vi "CRYCalibration.vi"(4 "O_Signal Type Old In":string[][](array[string]), 5 "Apply?":bool=TRUE, 6 "I_Signal Type Old In":string[][](array[string]), 7 "Hardware In":string, 8 "O_Calibrated Device Name Old In":string[][](array[string]), 9 "I_Calibrated Device Name Old In":string[][](array[string]), 10 "Calibration":T1 {"Calibration 2D"."Sens Curve"."Z data" items=["dB", "Lin"]; "Calibration 2D"."Sens Curve"."X data" items=["dB", "Lin"]; "Calibration 2D"."Sens Curve"."Y data" items=["dB", "Lin"]; "Calibration 2D"."Sens Curve"."Z dB ref" format="%.1f"; "Calibration 2D"."Sens Curve"."Z axis" items=["Log", "Lin"]; "Calibration 2D"."Sens Curve"."X dB ref" format="%.1f"; "Calibration 2D"."Sens Curve"."X axis" items=["Log", "Lin"]; "Calibration 2D"."Sens Curve"."Y axis" items=["Log", "Lin"]; "Calibration 2D"."Sens Curve"."Y dB ref" format="%.1f"; "Calibration 2D"."Sens Curve"."Curve"."z" format="%.2f"; "Calibration 2D"."Sens Curve"."Curve"."y" format="%.5p"; "Calibration 2D"."Sens Curve"."Curve"."x" format="%.2f"; "Calibration 2D"."EQ Curve"."Z data" items=["dB", "Lin"]; "Calibration 2D"."EQ Curve"."X data" items=["dB", "Lin"]; "Calibration 2D"."EQ Curve"."Y data" items=["dB", "Lin"]; "Calibration 2D"."EQ Curve"."Z dB ref" format="%.1f"; "Calibration 2D"."EQ Curve"."Z axis" items=["Log", "Lin"]; "Calibration 2D"."EQ Curve"."X dB ref" format="%.1f"; "Calibration 2D"."EQ Curve"."X axis" items=["Log", "Lin"]; "Calibration 2D"."EQ Curve"."Y axis" items=["Log", "Lin"]; "Calibration 2D"."EQ Curve"."Y dB ref" format="%.1f"; "Calibration 2D"."EQ Curve"."Curve"."z" format="%.2f"; "Calibration 2D"."EQ Curve"."Curve"."y" format="%.2f"; "Calibration 2D"."EQ Curve"."Curve"."x" format="%.2f"; "Calibration 2D"."Corr Curve"."Z data" items=["dB", "Lin"]; "Calibration 2D"."Corr Curve"."X data" items=["dB", "Lin"]; "Calibration 2D"."Corr Curve"."Y data" items=["dB", "Lin"]; "Calibration 2D"."Corr Curve"."Z dB ref" format="%.1f"; "Calibration 2D"."Corr Curve"."Z axis" items=["Log", "Lin"]; "Calibration 2D"."Corr Curve"."X dB ref" format="%.1f"; "Calibration 2D"."Corr Curve"."X axis" items=["Log", "Lin"]; "Calibration 2D"."Corr Curve"."Y axis" items=["Log", "Lin"]; "Calibration 2D"."Corr Curve"."Y dB ref" format="%.1f"; "Calibration 2D"."Corr Curve"."Curve"."z" format="%.2f"; "Calibration 2D"."Corr Curve"."Curve"."y" format="%.2f"; "Calibration 2D"."Corr Curve"."Curve"."x" format="%.2f"; "Calibration 2D"."Calibration"."EQ Step size" items=["R10", "R20", "R40", "R80", "User"]; "Calibration 2D"."Calibration"."Corr Step size" items=["R10", "R20", "R40", "R80", "User"]}, 11 "Proper VI No In":i32) -> (0 "O_Calibrated Device Name Out":string[][](array[string]), 1 "I_Calibrated Device Name Out":string[][](array[string]), 2 "O_Signal Type Out":string[][](array[string]), 3 "I_Signal Type Out":string[][](array[string]))   [LabVIEW 2013]
uses:
  Typedef Control/CRYCalibration All Cluster.ctl
  Typedef Control/CRYCalibration 2DCluster.ctl
  Typedef Control/CRYCalibration Cluster.ctl
  Typedef Control/CRYData Cluster.ctl
  CRYProject/CRYProject Editor Global.vi
panel:
  out "O_Signal Type Old In 2":string[][](array[string])
  out "I_Signal Type Old In 2":string[][](array[string])
  out "O_Name Out(Output Calibrated Name Out)":string[][](array[string])
  out "I_Name Out(Input Calibrated Name Out)":string[][](array[string])
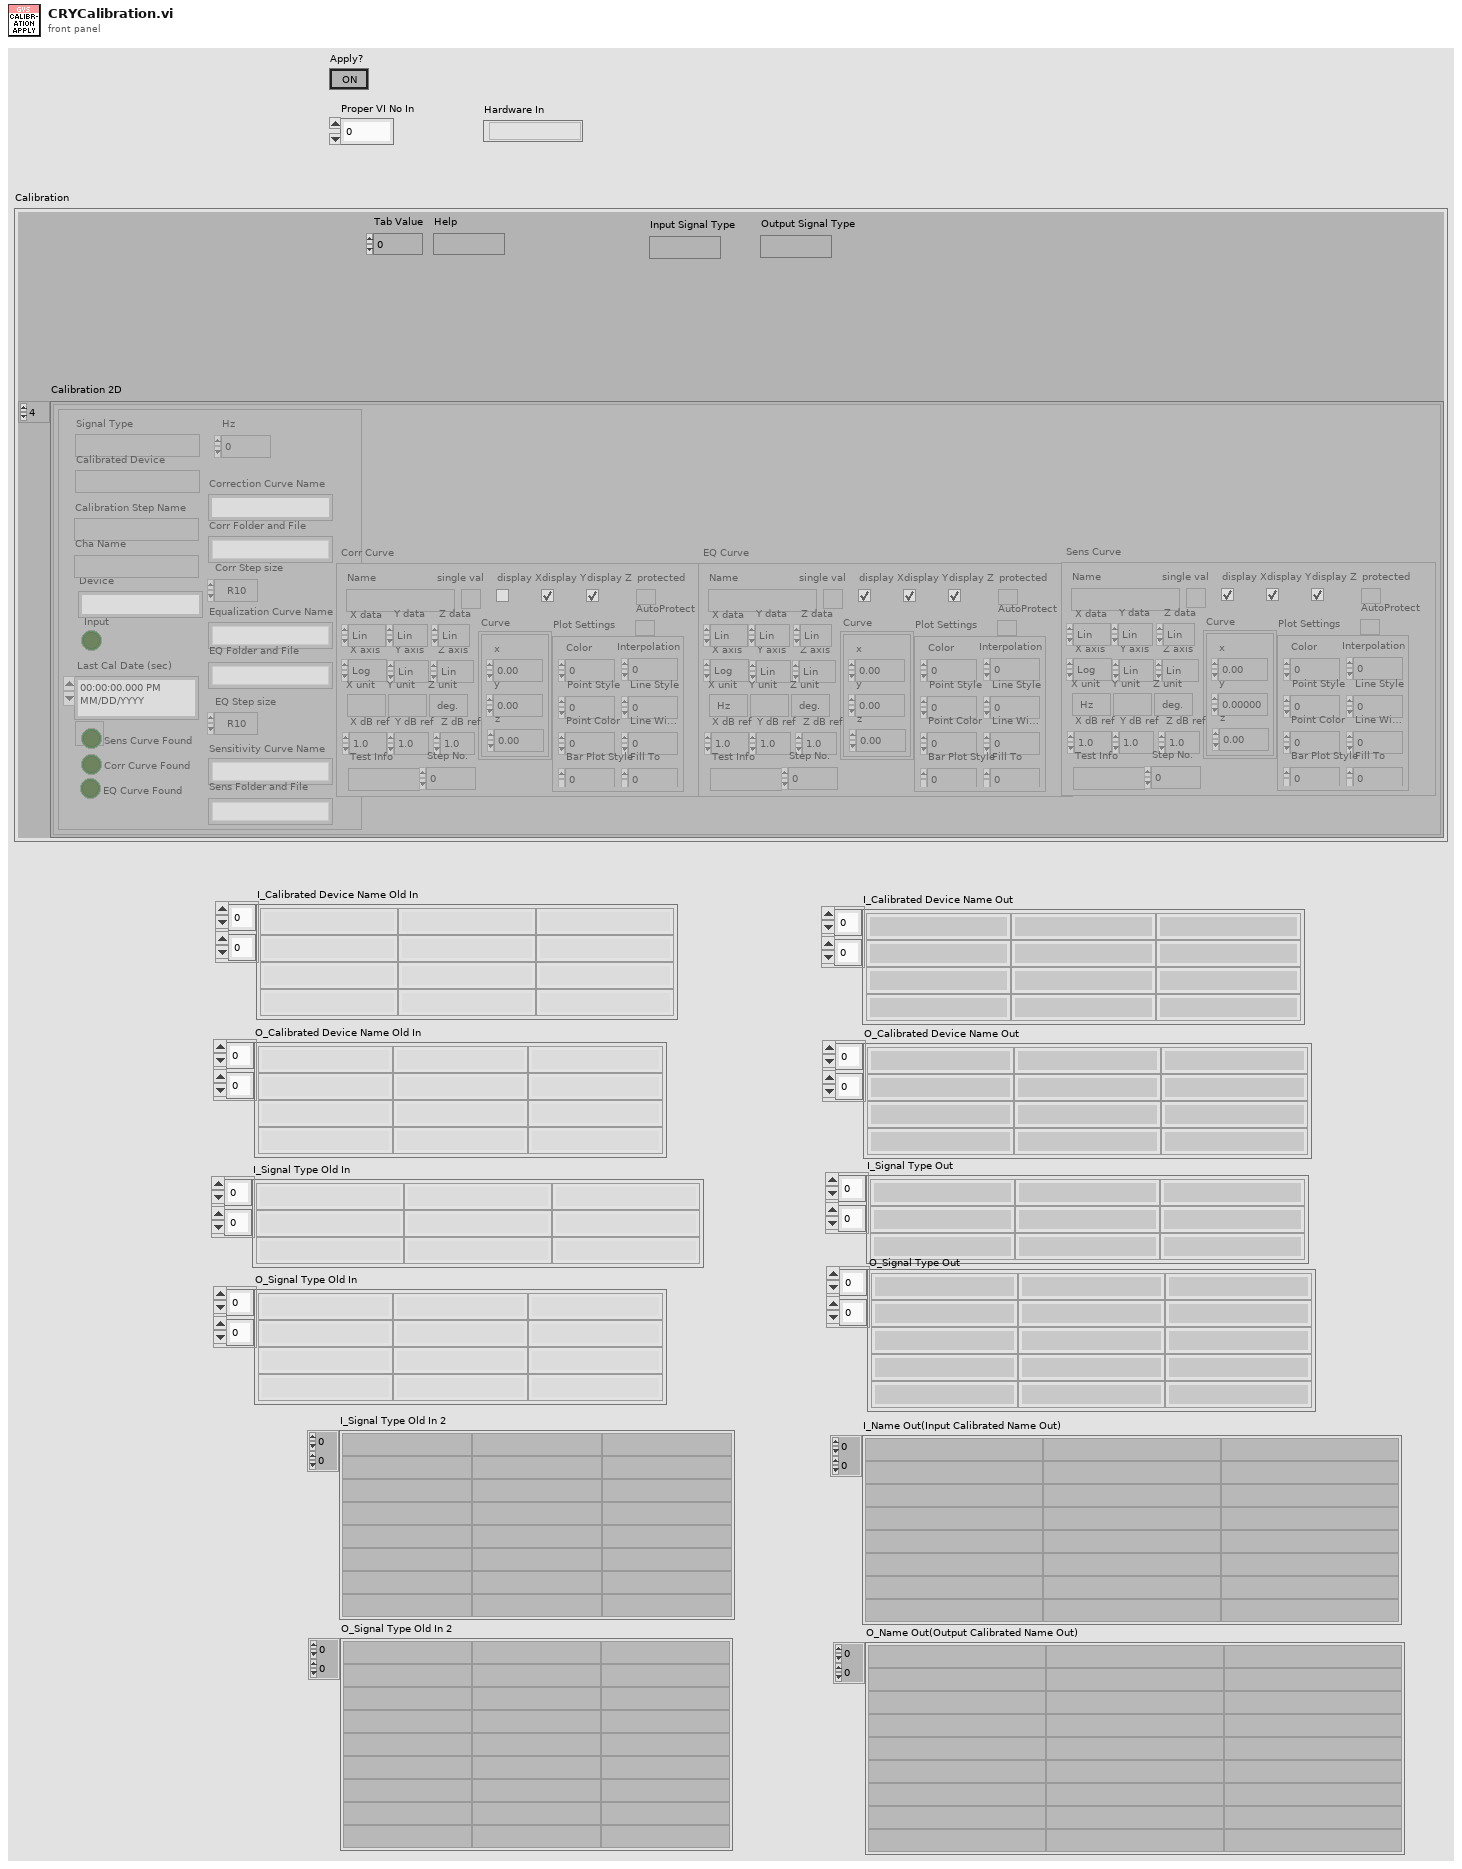
[diagram p1: front panel]
types:
  T1 = typedef "CRYCalibration All Cluster.ctl" = cluster{"Calibration 2D":T2[], "Help":string, "Tab Value":i32, "Input Signal Type":string, "Output Signal Type":string}
  T2 = typedef "CRYCalibration 2DCluster.ctl" = cluster{"Calibration":T3, "Corr Curve":T4, "EQ Curve":T4, "Sens Curve":T4}
  T3 = typedef "CRYCalibration Cluster.ctl" = cluster{"Calibration Step Name":string, "Device":string, "Correction Curve Name":string, "Equalization Curve Name":string, "Sensitivity Curve Name":string, "Corr Folder and File":string, "EQ Folder and File":string, "Sens Folder and File":string, "Corr Step size":u16, "EQ Step size":u16, "Input":bool, "Last Cal Date (sec)":timestamp, "Cha Name":string, "Corr Curve Found":bool, "EQ Curve Found":bool, "Sens Curve Found":bool, "Signal Type":string, "Calibrated Device":string, "Hz":u32}
  T4 = typedef "CRYData Cluster.ctl" = cluster{"Name":string, "Curve":cluster{"x":dbl, "y":dbl, "z":dbl}[], "X data":u16, "Y data":u16, "Z data":u16, "X axis":u16, "Y axis":u16, "Z axis":u16, "X unit":string, "Y unit":string, "Z unit":string, "X dB ref":dbl, "Y dB ref":dbl, "Z dB ref":dbl, "single val":bool, "protected":bool, "display X":bool, "display Y":bool, "display Z":bool, "Test Info":string, "Step No.":i32, "Plot Settings":cluster{"Color":u32, "Interpolation":u8, "Point Style":u8, "Line Style":u8, "Point Color":u32, "Line Width":u8, "Bar Plot Style":u8, "Fill To":i16}, "AutoProtect":bool}
  T5 = typedef "CRYStep.ctl" = cluster{"No.VI":i32, "Category":string, "StepName":string, "Seq setup flattened":string, "Comment":string, "Steps config.":bool[], "Jump config":i32[], "Start":dbl, "Increment":dbl, "Name":string, "Unit":string, "Y data":u16, "Y prefix":string, "Y dB ref":dbl, "Y unit":string, "Repeat State Array":cluster{"Start":dbl, "Increment":dbl, "Count":i32, "Num":i32}[]}
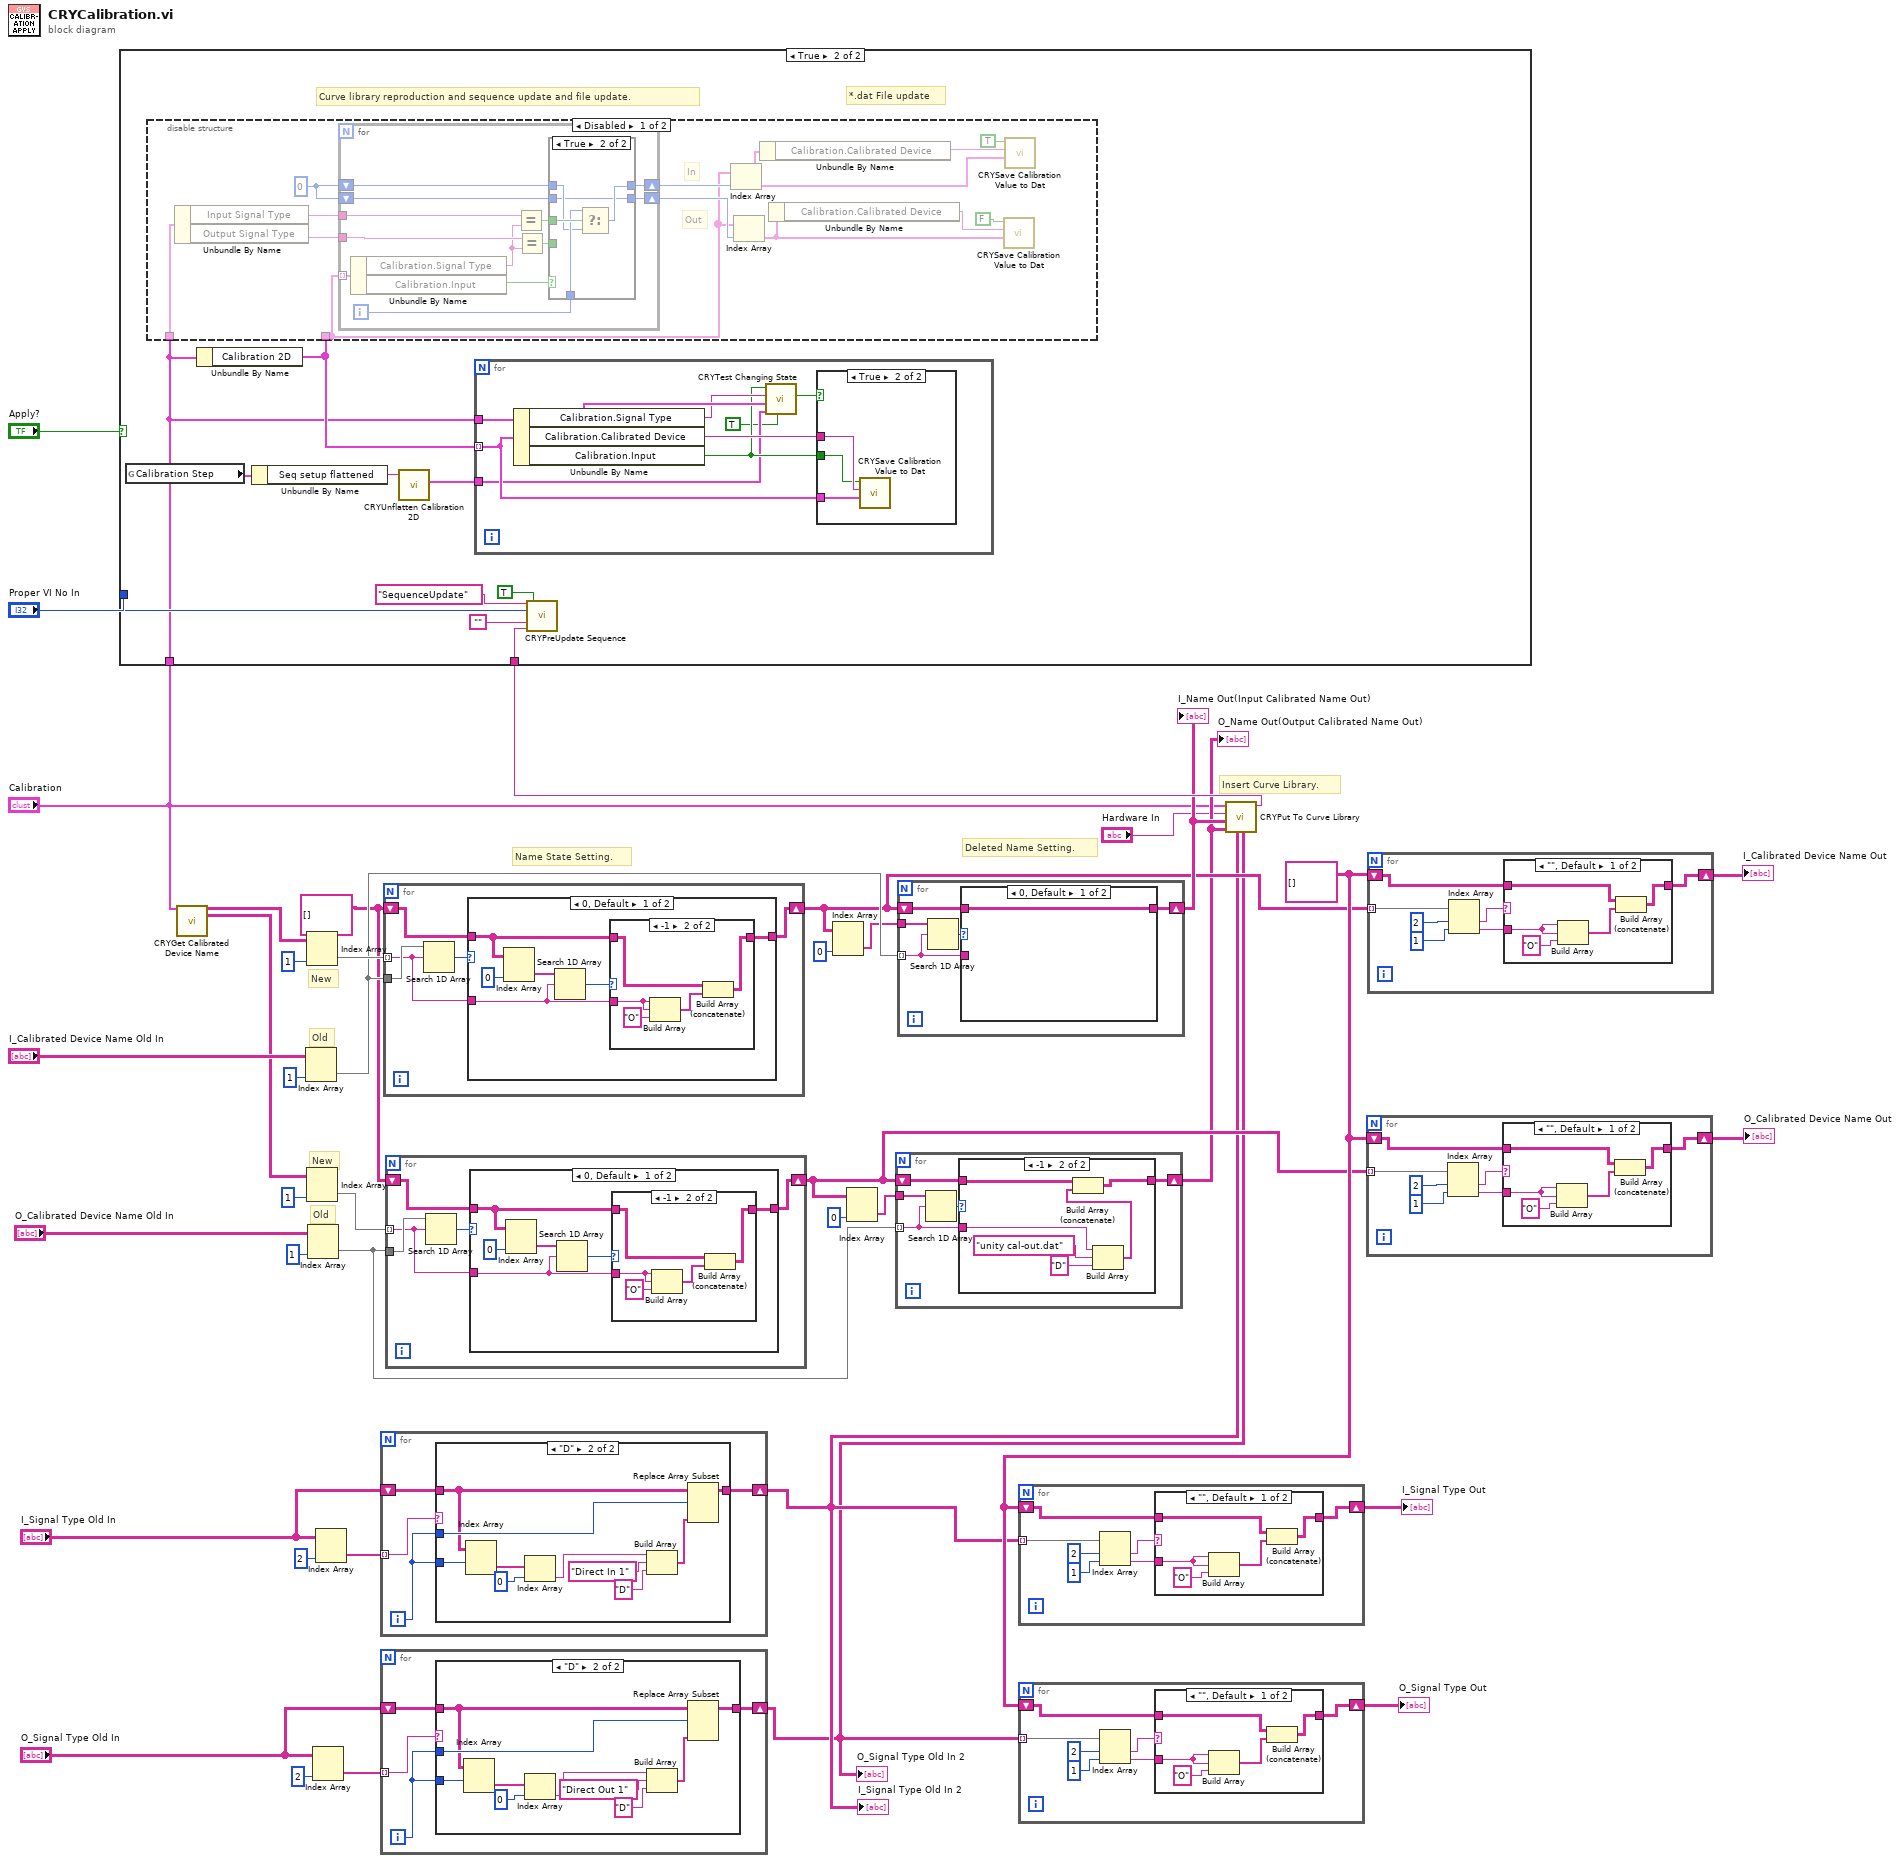
[diagram p0: block diagram]
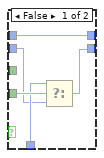
[diagram p3: hidden frame]
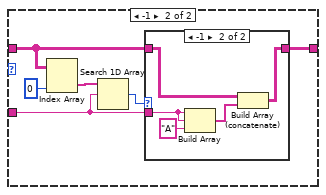
[diagram p8: hidden frame]
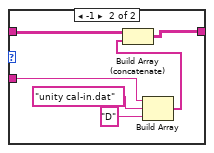
[diagram p16: hidden frame]
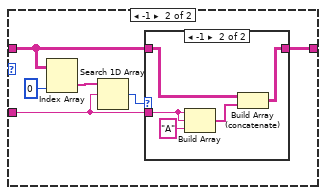
[diagram p18: hidden frame]
diagram:
  w12 = string[][] []
  w19 = string[][] []
  # "Old"
  # "New"
  # "Old"
  # "New"
  # "Deleted Name Setting."
  # "Name State Setting."
  # "Insert Curve Library."
  n1 = call "CRYGet Calibrated Device Name.vi"("Calibration"="Calibration") -> ("I_Name Out(Input Calibrated Name Out)"=w34:string[][], "O_Name Out(Output Calibrated Name Out)"=w31:string[][])  [unwired: 7 in, 6 out]
  n2 = Index Array(array="I_Calibrated Device Name Old In", index (col)=1 ("disabled index (col)")) -> (element=w29:string[])  [unwired: 1 in]
  n3 = Index Array(array=w34, index (col)=1 ("disabled index (col)")) -> (element=w30:string[])  [unwired: 1 in]
  n4 = Index Array(array=w31, index (col)=1 ("disabled index (col)")) -> (element=w11:string[])  [unwired: 1 in]
  n5 = Index Array(array="O_Calibrated Device Name Old In", index (col)=1 ("disabled index (col)")) -> (element=w9:string[])  [unwired: 1 in]
  n6 = Index Array(array="O_Signal Type Old In", index (col)=2 ("disabled index (col)")) -> (element=w22:string[])  [unwired: 1 in]
  n7 = Index Array(array="I_Signal Type Old In", index (col)=2 ("disabled index (col)")) -> (element=w23:string[])  [unwired: 1 in]
  n8 = for {
    tunnel: w23 -> [w43] mode=indexing
    shift-right: [w41] -> w5
    shift-left: "I_Signal Type Old In" -> [w42]
    i -> [w40]
    n9 = case shown="\"D\"" w43 {
      tunnel: [w44 w54] -> w41
      tunnel: w40 -> [_ w53]
      tunnel: w42 -> [w44 w52]
      tunnel: w40 -> [_ w51]
      frame "0", Default {
      }
      frame "D" {
        n10 = Index Array(array=w52, index (row)=w51) -> (element=w50:string[])  [unwired: 1 in]
        n11 = Index Array(array=w50, index=0) -> (element=w48:string)
        n12 = Build Array(w48, "Direct In 1" ("element"), "D" ("element")) -> (w45:string[])
        n13 = Replace Array Subset(array=w52, new element=w45, index (row)=w53) -> (w54:string[][])  [unwired: 1 in]
      }
    }
  }
  "I_Signal Type Old In 2" <- w5
  n14 = for {
    tunnel: w22 -> [w58] mode=indexing
    shift-right: [w56] -> w4
    shift-left: "O_Signal Type Old In" -> [w57]
    i -> [w55]
    n15 = case shown="\"D\"" w58 {
      tunnel: [w59 w69] -> w56
      tunnel: w55 -> [_ w68]
      tunnel: w57 -> [w59 w67]
      tunnel: w55 -> [_ w66]
      frame "0", Default {
      }
      frame "D" {
        n16 = Index Array(array=w67, index (row)=w66) -> (element=w60:string[])  [unwired: 1 in]
        n17 = Index Array(array=w60, index=0) -> (element=w64:string)
        n18 = Build Array(w64, "Direct Out 1" ("element"), "D" ("element")) -> (w61:string[])
        n19 = Replace Array Subset(array=w67, new element=w61, index (row)=w68) -> (w69:string[][])  [unwired: 1 in]
      }
    }
  }
  "O_Signal Type Old In 2" <- w4
  n20 = for {
    tunnel: w29 -> [w74]
    shift-right: [w70] -> w13
    shift-left: w12 -> [w72]
    tunnel: w30 -> [w71] mode=indexing
    n21 = Search 1D Array(1D array=w74, element=w71) -> (index of element=w73:i32)  [unwired: 1 in]
    n22 = case shown="0, Default" w73 {
      tunnel: w72 -> [w76 w91]
      tunnel: w71 -> [w77 w88]
      tunnel: [w75 w92] -> w70
      frame 0, Default {
        n23 = Index Array(array=w76, index (col)=0 ("disabled index (col)")) -> (element=w79:string[])  [unwired: 1 in]
        n24 = Search 1D Array(1D array=w79, element=w77) -> (index of element=w78:i32)  [unwired: 1 in]
        n25 = case shown="-1" w78 {
          tunnel: [w81 w84] -> w75
          tunnel: w76 -> [w81 w83]
          tunnel: w77 -> [_ w82]
          frame 0, Default {
          }
          frame -1 {
            n26 = Build Array(w82, w82, "O" ("element")) -> (w85:string[])
            n27 = Build Array (concatenate)(w83, w85) -> (w84:string[][])
          }
        }
      }
      frame -1 {
        n28 = Index Array(array=w91, index (col)=0 ("disabled index (col)")) -> (element=w89:string[])  [unwired: 1 in]
        n29 = Search 1D Array(1D array=w89, element=w88) -> (index of element=w87:i32)  [unwired: 1 in]
        n30 = case shown="-1" w87 {
          tunnel: [w93 w96] -> w92
          tunnel: w91 -> [w93 w95]
          tunnel: w88 -> [_ w94]
          frame 0, Default {
          }
          frame -1 {
            n31 = Build Array(w94, w94, "A" ("element")) -> (w97:string[])
            n32 = Build Array (concatenate)(w95, w97) -> (w96:string[][])
          }
        }
      }
    }
  }
  n33 = for {
    tunnel: w9 -> [w103]
    shift-right: [w99] -> w7
    shift-left: w12 -> [w101]
    tunnel: w11 -> [w100] mode=indexing
    n34 = Search 1D Array(1D array=w103, element=w100) -> (index of element=w102:i32)  [unwired: 1 in]
    n35 = case shown="0, Default" w102 {
      tunnel: w101 -> [w105 w120]
      tunnel: w100 -> [w106 w117]
      tunnel: [w104 w121] -> w99
      frame 0, Default {
        n36 = Index Array(array=w105, index (col)=0 ("disabled index (col)")) -> (element=w108:string[])  [unwired: 1 in]
        n37 = Search 1D Array(1D array=w108, element=w106) -> (index of element=w107:i32)  [unwired: 1 in]
        n38 = case shown="-1" w107 {
          tunnel: [w110 w113] -> w104
          tunnel: w105 -> [w110 w112]
          tunnel: w106 -> [_ w111]
          frame 0, Default {
          }
          frame -1 {
            n39 = Build Array(w111, w111, "O" ("element")) -> (w114:string[])
            n40 = Build Array (concatenate)(w112, w114) -> (w113:string[][])
          }
        }
      }
      frame -1 {
        n41 = Index Array(array=w120, index (col)=0 ("disabled index (col)")) -> (element=w118:string[])  [unwired: 1 in]
        n42 = Search 1D Array(1D array=w118, element=w117) -> (index of element=w116:i32)  [unwired: 1 in]
        n43 = case shown="-1" w116 {
          tunnel: [w122 w125] -> w121
          tunnel: w120 -> [w122 w124]
          tunnel: w117 -> [_ w123]
          frame 0, Default {
          }
          frame -1 {
            n44 = Build Array(w123, w123, "A" ("element")) -> (w126:string[])
            n45 = Build Array (concatenate)(w124, w126) -> (w125:string[][])
          }
        }
      }
    }
  }
  n46 = Index Array(array=w13, index (col)=0 ("disabled index (col)")) -> (element=w15:string[])  [unwired: 1 in]
  n47 = Index Array(array=w7, index (col)=0 ("disabled index (col)")) -> (element=w8:string[])  [unwired: 1 in]
  n48 = for {
    tunnel: w8 -> [w129]
    tunnel: w9 -> [w128] mode=indexing
    shift-right: [w131] -> w6
    shift-left: w7 -> [w132]
    n49 = Search 1D Array(1D array=w129, element=w128) -> (index of element=w130:i32)  [unwired: 1 in]
    n50 = case shown="-1" w130 {
      tunnel: w132 -> [w133 w139]
      tunnel: [w133 w138] -> w131
      tunnel: w128 -> [_ w135]
      frame 0, Default {
      }
      frame -1 {
        n51 = Build Array(w135, "unity cal-out.dat" ("element"), "D" ("element")) -> (w136:string[])
        n52 = Build Array (concatenate)(w139, w136) -> (w138:string[][])
      }
    }
  }
  "O_Name Out(Output Calibrated Name Out)" <- w6
  n53 = for {
    tunnel: w15 -> [w141]
    tunnel: w29 -> [w140] mode=indexing
    shift-right: [w143] -> w14
    shift-left: w13 -> [w144]
    n54 = Search 1D Array(1D array=w141, element=w140) -> (index of element=w142:i32)  [unwired: 1 in]
    n55 = case shown="0, Default" w142 {
      tunnel: w144 -> [w145 w151]
      tunnel: [w145 w150] -> w143
      tunnel: w140 -> [_ w147]
      frame 0, Default {
      }
      frame -1 {
        n56 = Build Array(w147, "unity cal-in.dat" ("element"), "D" ("element")) -> (w148:string[])
        n57 = Build Array (concatenate)(w151, w148) -> (w150:string[][])
      }
    }
  }
  "I_Name Out(Input Calibrated Name Out)" <- w14
  n58 = for {
    tunnel: w5 -> [w156] mode=indexing
    shift-right: [w152] -> w17
    shift-left: w19 -> [w153]
    n59 = Index Array(array=w156, index #1=2 ("index"), index #2=1 ("index")) -> (element #1=w154:string, element #2=w155:string)
    n60 = case shown="\"\", Default" w154 {
      tunnel: w155 -> [w162 _]
      tunnel: w153 -> [w161 w164]
      tunnel: [w159 w164] -> w152
      frame "", Default {
        n61 = Build Array(w162, w162, "O" ("element")) -> (w160:string[])
        n62 = Build Array (concatenate)(w161, w160) -> (w159:string[][])
      }
      frame "D" {
      }
    }
  }
  "I_Signal Type Out" <- w17
  n63 = for {
    tunnel: w4 -> [w169] mode=indexing
    shift-right: [w165] -> w18
    shift-left: w19 -> [w166]
    n64 = Index Array(array=w169, index #1=2 ("index"), index #2=1 ("index")) -> (element #1=w167:string, element #2=w168:string)
    n65 = case shown="\"\", Default" w167 {
      tunnel: w168 -> [w175 _]
      tunnel: w166 -> [w174 w177]
      tunnel: [w172 w177] -> w165
      frame "", Default {
        n66 = Build Array(w175, w175, "O" ("element")) -> (w173:string[])
        n67 = Build Array (concatenate)(w174, w173) -> (w172:string[][])
      }
      frame "D" {
      }
    }
  }
  "O_Signal Type Out" <- w18
  n68 = call "CRYPut To Curve Library.vi"("O_Signal Type In"=w4, "I_Signal Type In"=w5, "O_Calibrated Device Name In"=w6, "I_Calibrated Device Name In"=w14, "Hardware In"="Hardware In", "Calibration Step Cluster"="Calibration") -> ("Calibration flattened"=w26:string)  [unwired: 5 out]
  n69 = case shown="True" "Apply?" {
    tunnel: "Proper VI No In" -> [_ w184]
    tunnel: w26 -> [_ w183]
    tunnel: "Calibration" -> [_ w181]
    frame False {
    }
    frame True {
      # "*.dat File update"
      # "Curve library reproduction and sequence update and file update."
      n70 = global read "CRYProject Editor Global.vi" "Calibration Step"() -> (w180:T5)
      n71 = Unbundle By Name(w181) -> ("Calibration 2D"=w182:T2[])
      n72 = disable-structure shown="Disabled" {
        disable-tunnel: w181 -> [w200 _]
        disable-tunnel: w182 -> [w188 _]
        frame Disabled {
          w199 = 0
          # "Out"
          # "In"
          n73 = Unbundle By Name(w200) -> ("Input Signal Type"=w198:string, "Output Signal Type"=w197:string)
          n74 = for {
            tunnel: w188 -> [w212] mode=indexing
            shift-right: [w202] -> w196
            shift-left: w199 -> [w205]
            shift-right: [w201] -> w195
            shift-left: w199 -> [w204]
            tunnel: w198 -> [w210]
            tunnel: w197 -> [w209]
            i -> [w203]
            n75 = Unbundle By Name(w212) -> ("Calibration.Signal Type"=w208:string, "Calibration.Input"=w211:bool)
            n76 = Equal?(x=w210, y=w208) -> (x = y?=w207:bool)
            n77 = Equal?(x=w209, y=w208) -> (x = y?=w206:bool)
            n78 = case shown="True" w211 {
              tunnel: w207 -> [_ w222]
              tunnel: w206 -> [w217 _]
              tunnel: w205 -> [w213 w220]
              tunnel: w204 -> [w215 w218]
              tunnel: w203 -> [w216 w221]
              tunnel: [w213 w219] -> w202
              tunnel: [w214 w218] -> w201
              frame False {
                n79 = Select(t=w216, s=w217, f=w215) -> (s? t:f=w214:i32)
              }
              frame True {
                n80 = Select(t=w221, s=w222, f=w220) -> (s? t:f=w219:i32)
              }
            }
          }
          n81 = Index Array(array=w188, index=w196) -> (element=w189:T2)
          n82 = Index Array(array=w188, index=w195) -> (element=w191:T2)
          n83 = Unbundle By Name(w189) -> ("Calibration.Calibrated Device"=w190:string)
          n84 = Unbundle By Name(w191) -> ("Calibration.Calibrated Device"=w192:string)
          n85 = call "CRYSave Calibration Value to Dat.vi"("Calibration 2D Cluster"=w191, "Calibrated Device"=w192, "Input"=FALSE) -> ()  [unwired: 9 in]
          n86 = call "CRYSave Calibration Value to Dat.vi"("Calibration 2D Cluster"=w189, "Calibrated Device"=w190, "Input"=TRUE) -> ()  [unwired: 9 in]
        }
        frame Enabled {
        }
      }
      n87 = Unbundle By Name(w180) -> ("Seq setup flattened"=w179:string)
      n88 = call "CRYUnflatten Calibration 2D.vi"("Flattened Calibration"=w179) -> ("Calibration Step Out"=w178:T1)  [unwired: 8 in, 2 out]
      n89 = for {
        tunnel: w182 -> [w229] mode=indexing
        tunnel: w181 -> [w228]
        tunnel: w178 -> [w224]
        n90 = Unbundle By Name(w229) -> ("Calibration.Signal Type"=w227:string, "Calibration.Calibrated Device"=w230:string, "Calibration.Input"=w226:bool)
        n91 = call "CRYTest Changing State.vi"("Save?"=TRUE, "Origine Calibration"=w224, "New Calibration"=w228, "Signal Type"=w227, "In/Out?"=w226) -> ("Changed/Added"=w225:bool)  [unwired: 4 in, 2 out]
        n92 = case shown="True" w225 {
          tunnel: w230 -> [_ w233]
          tunnel: w229 -> [_ w231]
          tunnel: w226 -> [_ w232]
          frame False {
          }
          frame True {
            n93 = call "CRYSave Calibration Value to Dat.vi"("Calibration 2D Cluster"=w231, "Calibrated Device"=w233, "Input"=w232) -> ()  [unwired: 9 in]
          }
        }
      }
      n94 = call "CRYPreUpdate Sequence.vi"("EventName"="SequenceUpdate", "Proper VI No"=w184, "Project View Step Name Identifier Arg1"="", "Step flattened Arg2"=w183, "AllChangeFlg"=TRUE ("Name/Identifier")) -> ()  [unwired: 11 in]
    }
  }
  n95 = for {
    tunnel: w7 -> [w238] mode=indexing
    shift-right: [w234] -> w27
    shift-left: w19 -> [w235]
    n96 = Index Array(array=w238, index #1=2 ("index"), index #2=1 ("index")) -> (element #1=w236:string, element #2=w237:string)
    n97 = case shown="\"\", Default" w236 {
      tunnel: w237 -> [w244 _]
      tunnel: w235 -> [w243 w246]
      tunnel: [w241 w246] -> w234
      frame "", Default {
        n98 = Build Array(w244, w244, "O" ("element")) -> (w242:string[])
        n99 = Build Array (concatenate)(w243, w242) -> (w241:string[][])
      }
      frame "D" {
      }
    }
  }
  "O_Calibrated Device Name Out" <- w27
  n100 = for {
    tunnel: w13 -> [w251] mode=indexing
    shift-right: [w247] -> w28
    shift-left: w19 -> [w248]
    n101 = Index Array(array=w251, index #1=2 ("index"), index #2=1 ("index")) -> (element #1=w249:string, element #2=w250:string)
    n102 = case shown="\"\", Default" w249 {
      tunnel: w250 -> [w257 _]
      tunnel: w248 -> [w256 w259]
      tunnel: [w254 w259] -> w247
      frame "", Default {
        n103 = Build Array(w257, w257, "O" ("element")) -> (w255:string[])
        n104 = Build Array (concatenate)(w256, w255) -> (w254:string[][])
      }
      frame "D" {
      }
    }
  }
  "I_Calibrated Device Name Out" <- w28
